vi "BaseActions.vi"(8 "error in (no error)":errorcluster caption="entrée d'erreur (pas d'erreur)", 11 "DNLObjectIn":refnum<class "Tools.lvclass"> caption="DNLObject In") -> (0 "error out":errorcluster caption="sortie d'erreur", 3 "DNLObjectOut":refnum<class "Tools.lvclass">)   [LabVIEW 2019, in "Tools.lvclass"]
uses:
  Tools.lvclass
  C:/Programmes Labview/LabScanV1A/DevicesClass/BaseDevice/BaseDevice.lvclass
panel:
  out "Function":string
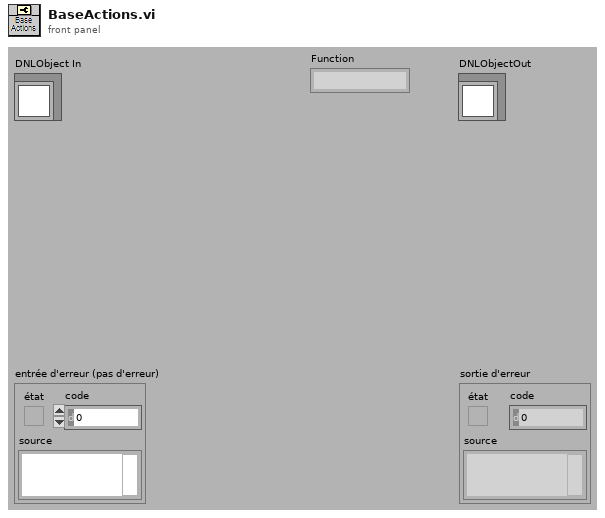
[diagram p1: front panel]
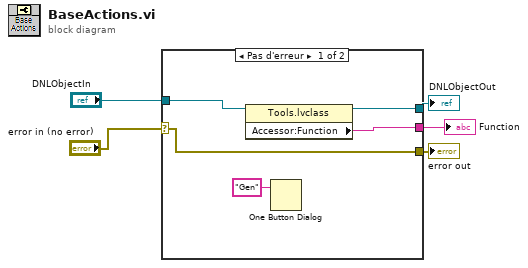
[diagram p0: block diagram]
diagram:
  n1 = case shown="Pas d'erreur" "error in (no error)" {
    selector: "error in (no error)" -> [w10 w11]
    tunnel: [w7 w12] -> w5
    tunnel: "DNLObjectIn" -> [w9 w12]
    tunnel: [w10 w11] -> w2
    tunnel: [w8 _] -> w1
    frame No Error {
      n2 = property class="Tools.lvclass"(reference=w9) -> (reference out=w7:refnum<class "Tools.lvclass">, "Accessor:Function"=w8:string)  [unwired: 1 in, 1 out]
      n3 = One Button Dialog(message="Gen") -> ()  [unwired: 1 in, 1 out]
    }
    frame Error {
    }
  }
  "error out" <- w2
  "DNLObjectOut" <- w5
  "Function" <- w1
